vi "CSM Application Running Log Example.vi"() -> ()   [LabVIEW 2017]
doc: "## CSM Application Running Log Example.vi\n\n### Overview\n\nDemonstrates how to use the CSM Logger VIs to implement global CSM event file logging.\n\n### Introduction\n\nThis example demonstrates how to use the CSM Logger VIs to implement global CSM event file logging. Use the CSM-Start File Logger VI, found under LabVIEW Palette -> CSM -> Addons -> Logger, to quickly implement global CSM event file logging.\n\nIn this example, two instances of the CSM-Start File Logger VI are placed in sequence, the log file path and name are manually set , and global rule filters are enabled for each instance separately. After running this example, you can locate and view the corresponding log files to deepen your understanding. If you add/call more CSM modules later, you do not need to change any code here to achieve logging functionality. In summary, a single high-level CSM Addon Logger VI is sufficient to quickly realize a global logging mechanism.\n\n### Steps\n\n- Step1: This is a simple CSM module named `RunningLogExample`.\n- Step2: Any button click will run into the \"API: Button Click\" state and broadcast a status change of the same name, with the button name as the parameter.\n- Step3: In `API: Button Click`, nothing needs to be done because the goal is to observe the log file.\n- Step4: After the program starts, two background logging threads for log files are launched. These logging threads will exit as the program exits.\n- Step5: After running the program, check the directory where the example VI is located for two log files.\n - Step5.1: `CSM Application Running Log Example.csmlog` records all logs.\n - Step5.2: `CSM Application Running Log Example.no-state.csmlog` records logs without state change records."
uses:
  user.lib/_NEVSTOP/Communicable State Machine(CSM)/addons/Logger/CSM File Logger Limit.ctl
  user.lib/_NEVSTOP/Communicable State Machine(CSM)/_Support/Typedef/_CSM_GlobalLog Filter Rules - v1.1.ctl
  user.lib/_NEVSTOP/Communicable State Machine(CSM)/_Support/Typedef/_CSM_GlobalLog_MSG_TYPE.ctl
  user.lib/_NEVSTOP/Communicable State Machine(CSM)/_Support/Typedef/_CSM_GlobalLog_STATE_TYPE.ctl
  user.lib/_NEVSTOP/Communicable State Machine(CSM)/_Support/GlobalEvent/GEvt-Convert Filter Rules - v1.1.vi
  user.lib/_NEVSTOP/Communicable State Machine(CSM)/AdvanceAPI/CSM - Break Down Multiple States String.vi
  user.lib/_NEVSTOP/Communicable State Machine(CSM)/AdvanceAPI/CSM - Compact Multiple States.vi
  user.lib/_NEVSTOP/Communicable State Machine(CSM)/AdvanceAPI/CSM - Revert Arguments-Safe String.vi
  user.lib/_NEVSTOP/Communicable State Machine(CSM)/AdvanceAPI/CSM - Make String Arguments Safe.vi
  user.lib/_NEVSTOP/Communicable State Machine(CSM)/AdvanceAPI/CSM - Keywords.vi
  user.lib/_NEVSTOP/Communicable State Machine(CSM)/_Support/GlobalEvent/LogFilter/SettingVIs/Set Global CSM Filter.vi
  user.lib/_NEVSTOP/Communicable State Machine(CSM)/_Support/GlobalEvent/LogFilter/SettingVIs/Set Global LogType Filter.vi
  user.lib/_NEVSTOP/Communicable State Machine(CSM)/_Support/GlobalEvent/LogFilter/SettingVIs/Set Global State Filter.vi
  user.lib/_NEVSTOP/Communicable State Machine(CSM)/_Support/GlobalEvent/LogFilter/SettingVIs/Set CSM LogType Filter.vi
  user.lib/_NEVSTOP/Communicable State Machine(CSM)/_Support/GlobalEvent/LogFilter/SettingVIs/Set CSM State Filter.vi
  user.lib/_NEVSTOP/Communicable State Machine(CSM)/_Support/GlobalEvent/LogFilter/SettingVIs/Set Global StateType Filter.vi
  user.lib/_NEVSTOP/Communicable State Machine(CSM)/_Support/GlobalEvent/LogFilter/SettingVIs/Set CSM StateType Filter.vi
  user.lib/_NEVSTOP/Communicable State Machine(CSM)/_Support/GlobalEvent/LogFilter/SettingVIs/Set Periodic Log Filter.vi
  user.lib/_NEVSTOP/Communicable State Machine(CSM)/_Shared/Trim Single-line Text.vi
  user.lib/_NEVSTOP/Communicable State Machine(CSM)/_Support/GlobalEvent/LogFilter/LogFilter.lvclass
  user.lib/_NEVSTOP/Communicable State Machine(CSM)/Communicable State Machine.lvlib
  user.lib/_NEVSTOP/Communicable State Machine(CSM)/addons/Logger/CSM File Logger.lvlib
panel:
  in  "Boolean 5":bool
  in  "Boolean 4":bool
  in  "Boolean 3":bool
  in  "Boolean 2":bool
  in  "Boolean 1":bool
  out "State History":string
  # "#CSM-Example Overview\n\nDemonstrates how to use the CSM Logger VIs to implement global CSM event file logging."
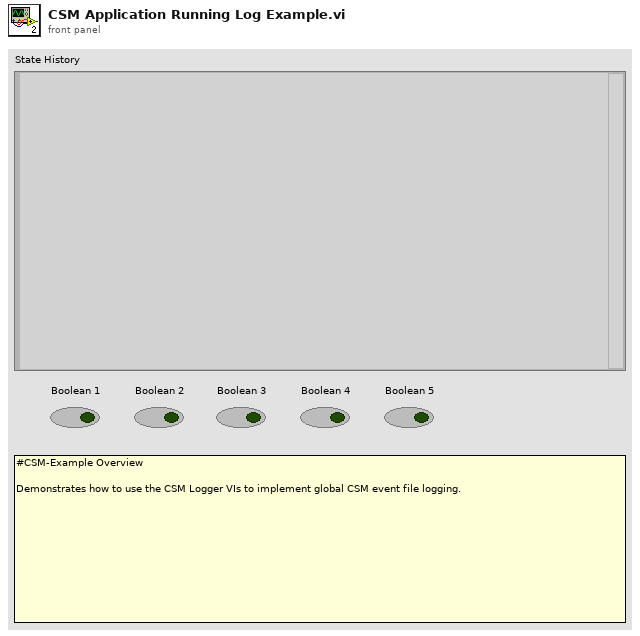
[diagram p1: front panel]
types:
  T1 = typedef "Communicable State Machine.lvlib/_CSM_GlobalLog Filter Rules - v1.1.ctl" = cluster{"Global":cluster{"CSM":string[], "LogType":T2[], "State":string[], "StateType":T3[]}, "CSM":cluster{"LogType":cluster{"CSM":string, "LogType":T2}[], "State":cluster{"CSM":string, "State":string}[], "StateType":cluster{"CSM":string, "LogType":T3}[]}, "PeriodicMessageFilter":cluster{"Enable":bool, "Threshold(#/s)":dbl, "CheckPeriod(s)":dbl}}
  T2 = typedef "Communicable State Machine.lvlib/_CSM_GlobalLog_MSG_TYPE.ctl" = enum16{"User Log", "State Change", "Status", "Interrupt", "Register", "Unregister", "Error Log", "Module Created", "Module Destroyed"}
  T3 = typedef "Communicable State Machine.lvlib/_CSM_GlobalLog_STATE_TYPE.ctl" = enum16{"State - Internal State", "State - External Message", "State - Response", "State - Complete"}
  T4 = typedef "CSM File Logger.lvlib/CSM File Logger Limit.ctl" = cluster{"file size (in bytes)":i64, "file num":i32}
  T5 = enum32{"Invalid", "Standard", "Closed", "Hidden", "Minimized", "Maximized"}
  T6 = enum32{"invalid app kind", "Development System", "Run Time System", "Student Edition", "Embedded LabVIEW", "Evaluation", "Custom"}
  T7 = typedef "Communicable State Machine.lvlib/_CSM_Response Source Message.ctl" = cluster{"‘State":string, "’Arguments":string, "’Error":errorcluster}
  T8 = cluster{"Current VI Reference":refnum<vi>, "Close Panel on Exit?":bool}
  T9 = cluster{"Core":cluster{"Current VI Reference":refnum<vi>, "Close Panel on Exit?":bool}, "Your Boolean data":bool, "Your string data":string}
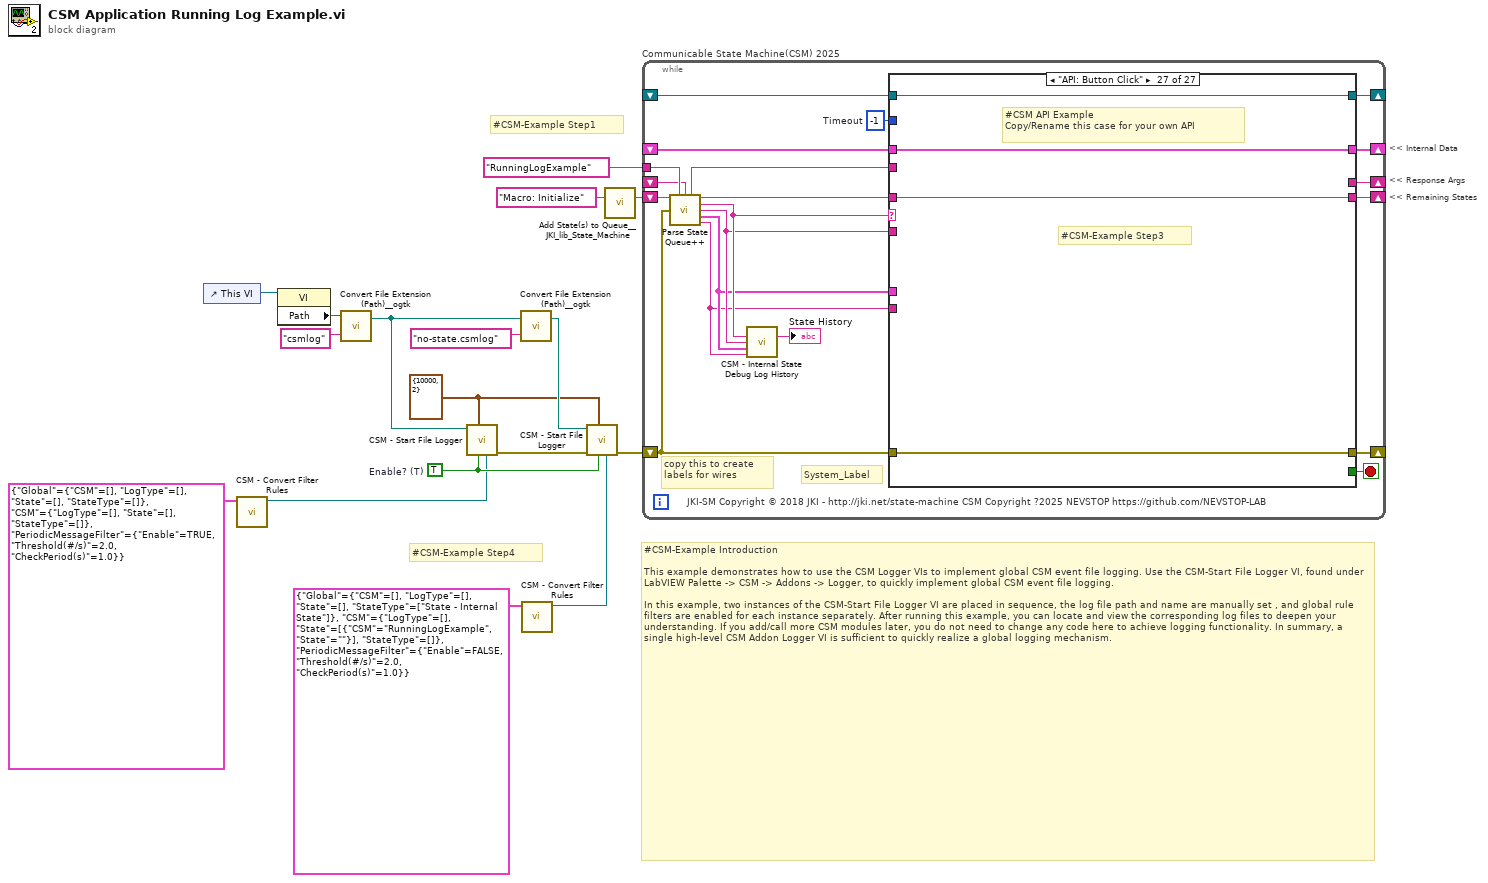
[diagram p0: block diagram]
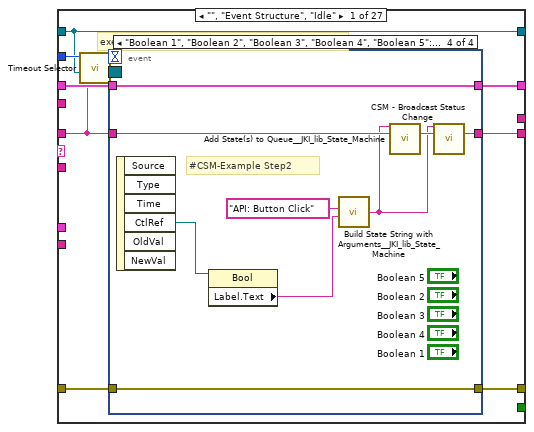
[diagram p2: hidden frame]
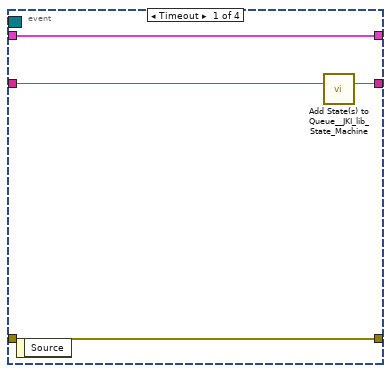
[diagram p3: hidden frame]
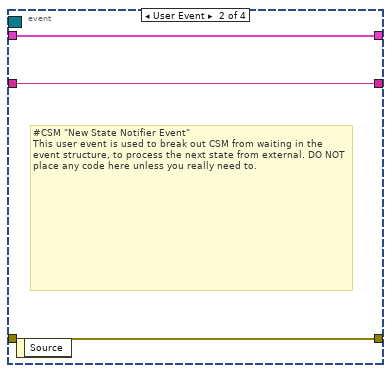
[diagram p4: hidden frame]
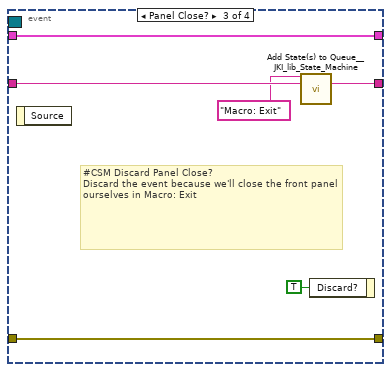
[diagram p5: hidden frame]
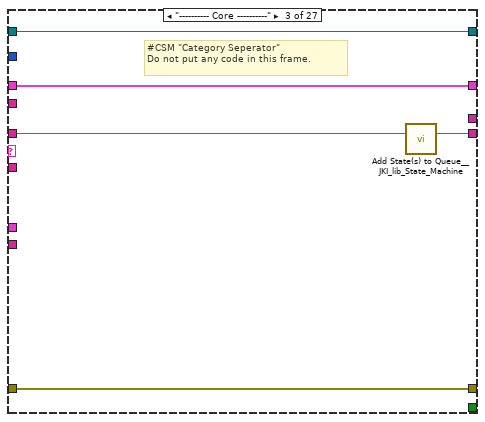
[diagram p7: hidden frame]
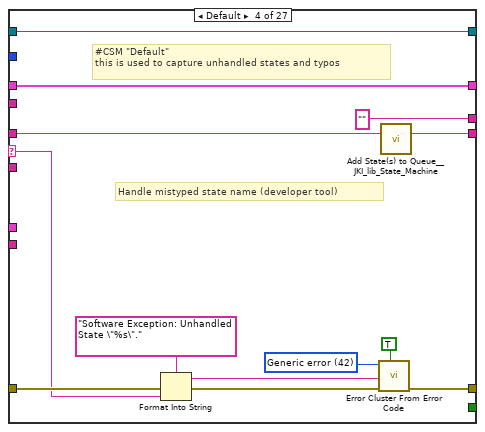
[diagram p8: hidden frame]
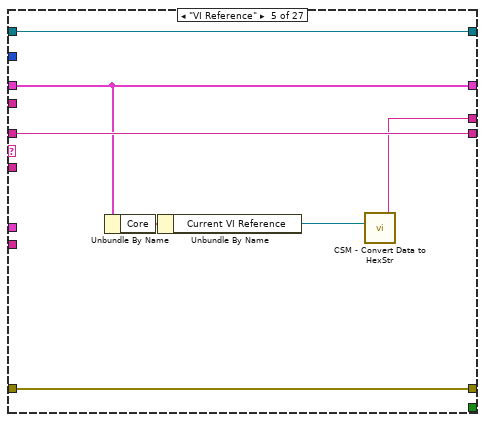
[diagram p9: hidden frame]
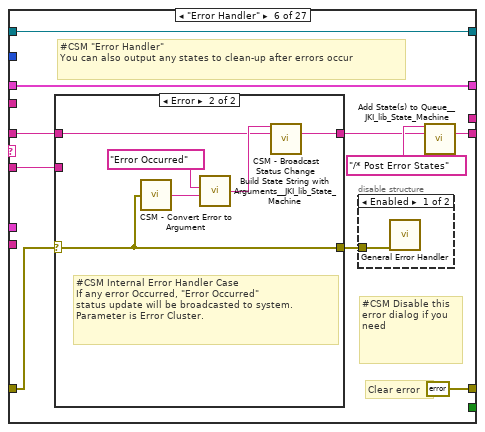
[diagram p10: hidden frame]
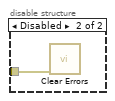
[diagram p11: hidden frame]
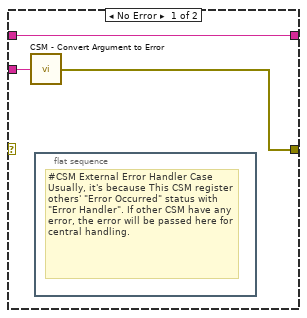
[diagram p12: hidden frame]
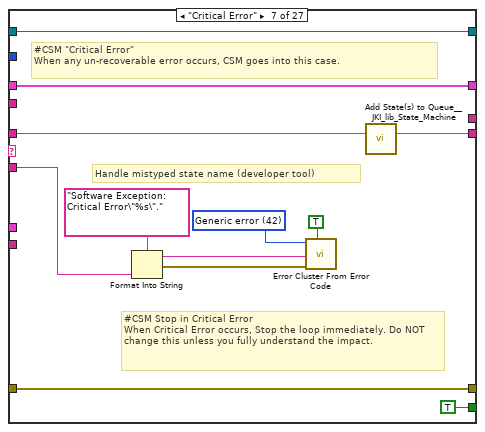
[diagram p13: hidden frame]
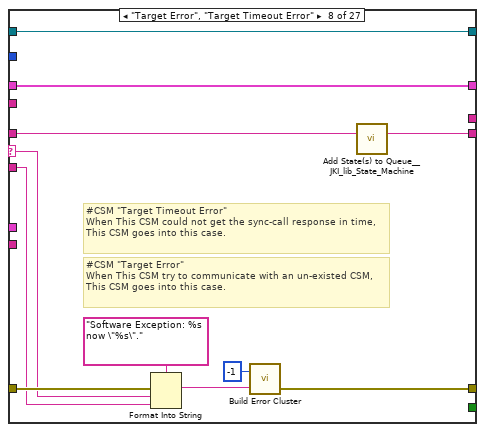
[diagram p14: hidden frame]
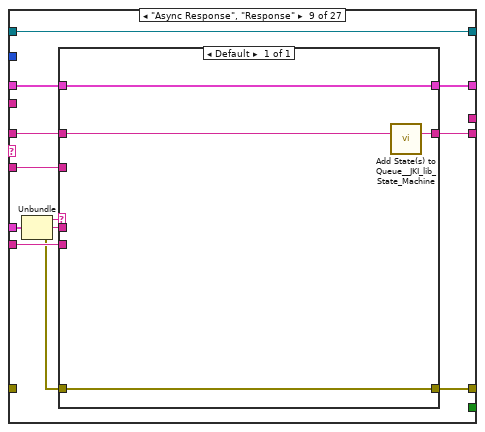
[diagram p15: hidden frame]
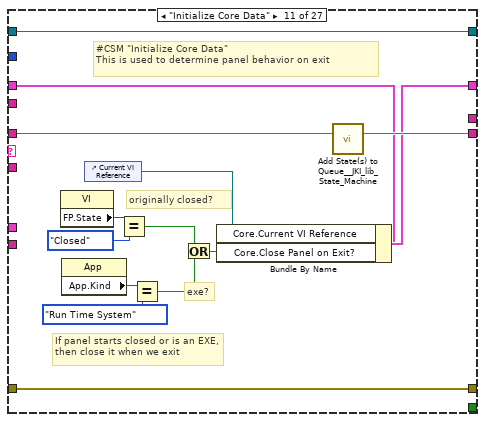
[diagram p17: hidden frame]
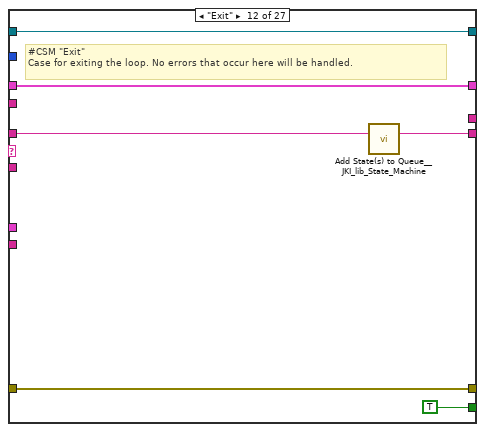
[diagram p18: hidden frame]
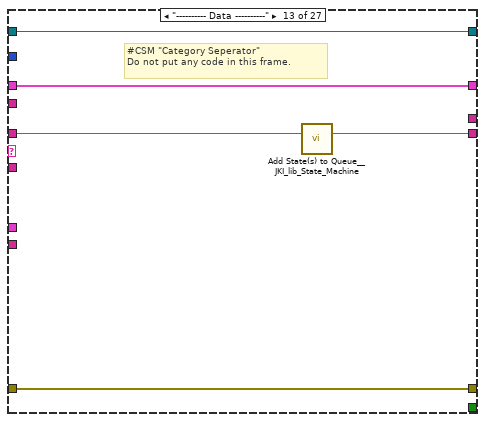
[diagram p19: hidden frame]
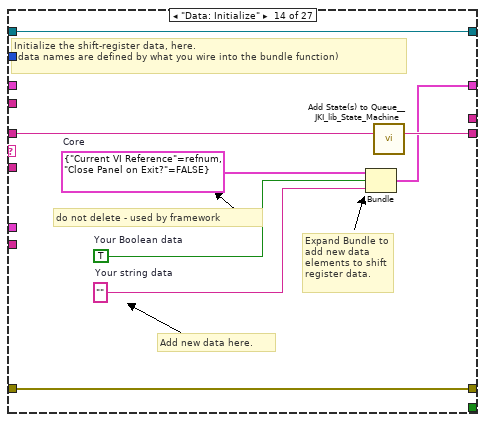
[diagram p20: hidden frame]
diagram:
  w5 = T4 {"file size (in bytes)"=10000, "file num"=2} ("log limit")
  w9 = TRUE  # Enable? (T)
  # "#CSM-Example Step4"
  # "#CSM-Example Step1"
  # "#CSM-Example Introduction\n\nThis example demonstrates how to use the CSM Logger VIs to implement global CSM event file logging. Use the CSM-Start File Logger VI, found under LabVIEW Palette -> CSM -> Addons -> Logger, to quickly implement global CSM event file logging.\n\nIn this example, two instances of the CSM-Start File Logger VI are placed in sequence, the log file path and name are manually set , and global rule filters are enabled for each instance separately. After running this example, you can locate and view the corresponding log files to deepen your understanding. If you add/call more CSM modules later, you do not need to change any code here to achieve logging functionality. In summary, a single high-level CSM Addon Logger VI is sufficient to quickly realize a global logging mechanism."
  # "<< Internal Data"
  # "<< Response Args"
  # "<< Remaining States"
  n1 = control-ref of="This VI"() -> (w13:refnum<vi>)
  n2 = call-poly "CSM - Convert Filter Rules.vi"("Rules-v1"=T1 {"Global"={"CSM"=[], "LogType"=[], "State"=[], "StateType"=[]}, "CSM"={"LogType"=[], "State"=[], "StateType"=[]}, "PeriodicMessageFilter"={"Enable"=TRUE, "Threshold(#/s)"=2.0, "CheckPeriod(s)"=1.0}}) -> ("GlobalLogFilter"=w1:refnum<class "LogFilter.lvclass">)  [unwired: 10 in]
  n3 = property class="VI"(reference=w13) -> ("Path"=w12:path)  [unwired: 1 in, 2 out]
  n4 = call "Convert File Extension (Path)__ogtk.vi"("New Ending (None)"="csmlog" ("new ending (none)"), "File Name"=w12) -> ("New Filename"=w7:path)  [unwired: 1 out]
  n5 = call "CSM - Start File Logger.vi"("Filter Rules"=w1, "Enable? (T)"=w9, "Log Limit"=w5, "Log File Path"=w7) -> ("error out"=w10:errorcluster)  [unwired: 5 in, 2 out]
  n6 = call "Convert File Extension (Path)__ogtk.vi"("New Ending (None)"="no-state.csmlog" ("new ending (none)"), "File Name"=w7) -> ("New Filename"=w6:path)  [unwired: 1 out]
  n7 = call-poly "CSM - Convert Filter Rules.vi"("Rules-v1"=T1 {"Global"={"CSM"=[], "LogType"=[], "State"=[], "StateType"=[enum."State - Internal State"]}, "CSM"={"LogType"=[], "State"=[{"CSM"="RunningLogExample", "State"=""}], "StateType"=[]}, "PeriodicMessageFilter"={"Enable"=FALSE, "Threshold(#/s)"=2.0, "CheckPeriod(s)"=1.0}}) -> ("GlobalLogFilter"=w4:refnum<class "LogFilter.lvclass">)  [unwired: 10 in]
  n8 = call "CSM - Start File Logger.vi"("Filter Rules"=w4, "Enable? (T)"=w9, "Log Limit"=w5, "Error In"=w10, "Log File Path"=w6) -> ("error out"=w14:errorcluster)  [unwired: 4 in, 2 out]
  n9 = call <vilib>:"Add State(s) to Queue__JKI_lib_State_Machine.vi"("State(s) in (\"\")"="Macro: Initialize" ("Init State(\"Macro: Initialize\")")) -> ("States Out"=w15:string)  [unwired: 14 in]
  n10 = while "Communicable State Machine(CSM) 2025" {
    shift-right: [w32] -> _
    shift-left: _ -> [w31]
    shift-right: [w35] -> _
    shift-left: w14 -> [w29]
    shift-right: [w34] -> _
    shift-left: w15 -> [w36]
    tunnel: "RunningLogExample" ("Name (\"\" to Use UUID)") -> [w25]
    shift-right: [w28] -> _
    shift-left: _ -> [w19]
    shift-right: [w27] -> _
    shift-left: _ -> [w26]
    stop <- w33 stop-if-true
    w30 = -1  # Timeout
    # "copy this to create labels for wires"
    # "System_Label"
    # "JKI-SM Copyright © 2018 JKI - http://jki.net/state-machine CSM Copyright ?2025 NEVSTOP https://github.com/NEVSTOP-LAB"
    n11 = call "Parse State Queue++.vi"("State Queue"=w36, "Name (\"\" to Use UUID)"=w25, "Response Arguments"=w19, "Previous Error"=w29) -> ("Name Used"=w20:string, "Remaining States"=w37:string, "Current State"=w24:string, "Arguments"=w23:string, "Additional Information"=w22:T7, "Source CSM"=w21:string)  [unwired: 6 in]
    n12 = call "CSM - Internal State Debug Log History.vi"("State"=w24, "Arguments (\"\")"=w23, ">> Response Source Message >>"=w22, "Source (\"\")"=w21) -> ("Debug Log"=→"State History":string)  [unwired: 11 in]
    n13 = case shown="\"API: Button Click\"" w24 {
      selector: w24 -> [_ _ _ w80 _ _ _ w134 _ _ _ _ _ _ _ _ _ _ _ _ _ _ _ _ _ _ _]
      tunnel: w37 -> [w38 w71 w77 w84 w96 w102 w128 w136 w147 w160 w175 w181 w186 w194 w201 w206 w213 w217 w223 w228 w235 w251 w321 w327 w339 w342 w346]
      tunnel: w23 -> [_ _ _ _ _ w101 w121 w135 w146 _ _ _ _ _ _ _ _ _ _ _ w230 w245 _ _ _ _ _]
      tunnel: w31 -> [w45 w70 w74 w82 w95 w106 w129 w138 w149 w159 w168 w179 w183 _ w196 w203 w212 w216 w220 w226 w233 w247 w318 w324 w336 w341 w345]
      tunnel: [w44 w72 w75 w86 w97 errorcluster {"status"=FALSE, "code"=0, "source"=""} ("error out") w130 w132 w152 w161 w172 w178 w184 w191 w197 w204 w207 w215 w221 w225 w231 w248 w319 w325 w337 w343 w347] -> w35
      tunnel: w29 -> [w43 w72 w75 w85 w97 w103 w130 w140 _ w161 w172 w178 w184 w191 w198 w204 _ w218 w221 w225 w232 w249 w319 w325 w337 w343 w347]
      tunnel: [w46 w71 w76 w83 w96 w98 w127 w139 w148 w160 w174 w180 w185 w193 w200 w205 w213 w217 w222 w227 w234 w250 w320 w326 w338 w342 w346] -> w34
      tunnel: [_ _ _ _ _ _ TRUE _ _ _ _ TRUE _ _ _ _ _ _ _ _ _ _ _ _ _ _ _] -> w33
      tunnel: [w42 w70 w74 w82 w95 w106 w129 w138 w150 w159 w173 w179 w183 w192 w196 w203 w212 w216 w220 w226 w233 w247 w318 w324 w336 w341 w345] -> w32
      tunnel: w30 -> [w41 _ _ _ _ _ _ _ _ _ _ _ _ _ _ _ _ _ _ _ _ _ _ _ _ _ _]
      tunnel: w21 -> [_ _ _ _ _ _ _ _ w144 _ _ _ _ _ _ _ _ _ _ _ _ _ _ _ _ _ _]
      tunnel: w22 -> [_ _ _ _ _ _ _ _ w151 _ _ _ _ _ _ _ _ _ _ _ _ _ _ _ _ _ _]
      tunnel: [_ _ _ "" w91 _ _ _ _ _ _ _ _ _ _ _ _ _ _ _ _ _ _ _ _ _ _] -> w28
      tunnel: [w40 w69 w73 w78 w94 w105 w119 w137 w153 w158 w162 w176 w182 w187 w195 w202 w211 w214 w219 w224 w229 w244 w317 w322 w329 w340 w344] -> w27
      tunnel: w26 -> [w40 w69 w73 w78 w94 w105 w119 w137 w153 w158 w162 w176 w182 w187 w195 w202 _ w214 w219 w224 w229 w244 w317 w322 w329 w340 w344]
      tunnel: w20 -> [_ _ _ _ _ _ _ _ _ _ _ _ _ _ _ _ w210 _ _ _ _ _ _ _ _ _ _]
      frame "", "Event Structure", "Idle" {
        # "executes when the state queue is empty"
        n14 = call "Timeout Selector.vi"("Remaining States"=w38, "Timeout Expected"=w41) -> ("Timeout"=w39:i32)  [unwired: 5 in]
        n15 = event shown="[3] \"Boolean 1\", \"Boolean 2\", \"Boolean 3\", \"Boolean 4\", \"Boolean 5\": Value Change" {
          selector: w40 -> [_ _ _ _]
          dyn-events: _ -> [_ _ _ _]
          timeout: w39 -> [_ _ _ _]
          tunnel: w38 -> [w50 w52 w59 w66]
          tunnel: [w49 w52 w58 w61] -> w46
          tunnel: w45 -> [w47 w53 w56 w67]
          tunnel: [w48 w51 w57 w68] -> w44
          tunnel: w43 -> [w48 w51 w57 w68]
          tunnel: [w47 w53 w56 w67] -> w42
          event Timeout {
            n16 = event-data() -> ()  [unwired: 1 in, 1 out]
            n17 = call <vilib>:"Add State(s) to Queue__JKI_lib_State_Machine.vi"("State(s) in (\"\")"=w50) -> ("States Out"=w49:string)  [unwired: 14 in]
          }
          event User Event {
            # "#CSM \"New State Notifier Event\"\nThis user event is used to break out CSM from waiting in the event structure, to process the next state from external. DO NOT place any code here unless you really need to."
            n18 = event-data() -> ()  [unwired: 1 in, 1 out]
          }
          event Panel Close? {
            # "#CSM Discard Panel Close?\nDiscard the event because we'll close the front panel ourselves in Macro: Exit"
            n19 = event-data() -> ()  [unwired: 1 in, 1 out]
            n20 = call <vilib>:"Add State(s) to Queue__JKI_lib_State_Machine.vi"("State(s) in Front (\"\")"="Macro: Exit", "State(s) in (\"\")"=w59) -> ("States Out"=w58:string)  [unwired: 13 in]
            n21 = event-data("Discard?"=TRUE) -> ()  [unwired: 1 in, 1 out]
          }
          event "Boolean 1", "Boolean 2", "Boolean 3", "Boolean 4", "Boolean 5": Value Change {
            # "#CSM-Example Step2"
            n22 = event-data() -> ("CtlRef"=w63:refnum<vi>)  [unwired: 1 in, 5 out]
            n23 = property class="Bool"(reference=w63) -> ("Label.Text"=w62:string)  [unwired: 1 in, 2 out]
            n24 = call <vilib>:"Build State String with Arguments__JKI_lib_State_Machine.vi"("Arguments (\"\")"=w62, "State"="API: Button Click") -> ("State with Arguments"=w60:string)  [unwired: 4 in]
            n25 = call <vilib>:"Add State(s) to Queue__JKI_lib_State_Machine.vi"("State(s) in Front (\"\")"=w60, "State(s) in (\"\")"=w66) -> ("States Out"=w65:string)  [unwired: 13 in]
            n26 = call "CSM - Broadcast Status Change.vi"("Status With Arguments"=w60, "State Queue"=w65) -> ("Remaining States"=w61:string)  [unwired: 13 in]
          }
        }
      }
      frame "CSM Documentation" {
        # "#CSM README FIRST\n\nCSM is a LabVIEW application framework that builds upon JKI State Machine (JKISM). It follows the pattern of JKISM and extends the keywords to describe message communication between CSM modules, including concepts such as Sync-Message, Async-Message, Subscription/Unsubscription of status - essential elements for creating reusable code modules. For more information, please visit the CSM wiki: https://github.com/NEVSTOP-LAB/JKI-State-Machine-Plus-Plus/wiki\n\nFor instructions on JKI State Machine, visit: http://jki.net/state-machine/\nFor information about CSM, visit: https://github.com/NEVSTOP-LAB"
        # "#CSM \"Documentation\"\nCase for holding CSM Documenation"
      }
      frame "---------- Core ----------" {
        # "#CSM \"Category Seperator\"\nDo not put any code in this frame."
        n27 = call <vilib>:"Add State(s) to Queue__JKI_lib_State_Machine.vi"("State(s) in (\"\")"=w77) -> ("States Out"=w76:string)  [unwired: 14 in]
      }
      frame Default {
        w89 = 42 items=["No error", "Argument error", "Memory is full", "Out of zone", "End of file", "File already open", "Generic file I/O error", "File not found", "File permission error", "Disk is full", "Duplicate path", "Too many files open", "System feature not enabled", "Resource file not found", "Cannot add resource", "Resource not found", "Image not found", "Image memory error", "Pen does not exist", "Config type invalid", "Config token not found", "Config parse error", "Config memory error", "Bad external code format", "Bad external code offset", "External code not present", "Null window", "Destroy window error", "Null menu", "Print aborted", "Bad print record", "Print driver error", "Windows error during printing", "Memory error during printing", "Print dialog error", "Generic print error", "Invalid device refnum", "Device not found", "Device parameter error", "Device unit error", "Cannot open device", "Device call aborted", "Generic error", "Cancelled by user", "Object ID too low", "Object ID too high", "Object not in heap", "Unknown heap", "Unknown object (invalid DefProc)", "Unknown object (DefProc not in table)", "Message out of range", "Invalid (null) method", "Unknown message", "Manager call not supported", "Bad address", "Network operation in progress", "Network operation timed out", "Connection is busy", "Network attribute not supported", "Network error", "Address in use", "System out of memory", "Connection aborted", "Connection refused", "Not connected", "Already connected", "Connection closed", "Initialization error (interapplication manager)", "Bad occurrence", "Wait on unbound occurrence handler", "Occurrence queue overflow", "Datalog type conflict", "Unused", "Unrecognized type (interapplication manager)", "Memory corrupt", "Failed to make temporary DLL", "Old CIN version", "Drag socket not found", "Failed to load drop-object", "Failed to register OLE object", "Failed to release OLE object", "Format specifier type mismatch", "Unknown format specifier", "Too few format specifiers", "Too many format specifiers", "Scan failed", "Newer CIN version", "Error converting to variant", "Runtime menu error", "Password tampered", "Variant attribute not found", "Incompatible variant data type", "Event data is not available", "Event Store is not present", "Occurrence is not found", "Event Queue is not created", "Event info is not available", "Refnum passed is NULL", "Error retrieving Class GUID", "Error retrieving CoClass GUID", "Error retrieving TypeLib GUID.", "Bad built application magic bytes.", "Specific driver is different from the specific driver associated with the Logical Name.", "There is no session opened to the class driver.", "Max Error", "MAX - Error with config objects", "MAX - Error loading configuration", "MAX - Group not supported"]
        # "#CSM \"Default\"\nthis is used to capture unhandled states and typos"
        # "Handle mistyped state name (developer tool)"
        n28 = Format Into String(format string="Software Exception: Unhandled State \"%s\"." ("message"), error in=w85, w80) -> (resulting string=w88:string, error out=w87:errorcluster)  [unwired: 1 in]
        n29 = call <vilib>:"Error Cluster From Error Code.vi"("show call chain? (False)"=TRUE, "error in (no error)"=w87, "error message (\"\")"=w88, "error code (0)"=w89) -> ("error out"=w86:errorcluster)  [unwired: 5 in]
        n30 = call <vilib>:"Add State(s) to Queue__JKI_lib_State_Machine.vi"("State(s) in (\"\")"=w84) -> ("States Out"=w83:string)  [unwired: 14 in]
      }
      frame "VI Reference" {
        n31 = Unbundle By Name(w95) -> ("Core"=w93:T8)
        n32 = Unbundle By Name(w93) -> ("Current VI Reference"=w92:refnum<vi>)
        n33 = call "CSM - Convert Data to HexStr.vi"("Variant"=w92) -> ("HEX String (0-9,A-F)"=w91:string)  [unwired: 8 in]
      }
      frame "Error Handler" {
        # "#CSM Disable this error dialog if you need"
        # "#CSM \"Error Handler\"\nYou can also output any states to clean-up after errors occur"
        # "Clear error"
        n34 = case shown="Error" w103 {
          selector: w103 -> [_ w113]
          tunnel: [w112 w115] -> w99
          tunnel: w102 -> [w112 w114]
          tunnel: w101 -> [w111 _]
          tunnel: [w110 w113] -> w104
          frame No Error {
            n35 = call "CSM - Convert Argument to Error.vi"("Argument"=w111) -> ("Error"=w110:errorcluster)  [unwired: 4 in]
            n36 = flat-sequence {
              frame #0 {
                # "#CSM External Error Handler Case\nUsually, it's because This CSM register others' \"Error Occurred\" status with \"Error Handler\". If other CSM have any error, the error will be passed here for central handling."
              }
            }
          }
          frame Error {
            # "#CSM Internal Error Handler Case \nIf any error Occurred, \"Error Occurred\" \nstatus update will be broadcasted to system.\nParameter is Error Cluster."
            n37 = call "CSM - Convert Error to Argument.vi"("Error"=w113) -> ("Argument"=w117:string)  [unwired: 4 in]
            n38 = call <vilib>:"Build State String with Arguments__JKI_lib_State_Machine.vi"("Arguments (\"\")"=w117, "State"="Error Occurred" ("Status with Arguments")) -> ("State with Arguments"=w116:string)  [unwired: 4 in]
            n39 = call "CSM - Broadcast Status Change.vi"("Status With Arguments"=w116, "State Queue"=w114) -> ("Remaining States"=w115:string)  [unwired: 13 in]
          }
        }
        n40 = disable-structure shown="Enabled" {
          disable-tunnel: w104 -> [w108 w109]
          frame Enabled {
            n41 = call <vilib>:"General Error Handler.vi"("error in (no error)"=w108) -> ()  [unwired: 10 in, 5 out]
          }
          frame Disabled {
            n42 = call <vilib>:"Clear Errors.vi"("error in (no error)"=w109) -> ()  [unwired: 5 in, 2 out]
          }
        }
        n43 = call <vilib>:"Add State(s) to Queue__JKI_lib_State_Machine.vi"("State(s) in Front (\"\")"="/* Post Error States", "State(s) in (\"\")"=w99) -> ("States Out"=w98:string)  [unwired: 13 in]
      }
      frame "Critical Error" {
        w125 = 42 items=["No error", "Argument error", "Memory is full", "Out of zone", "End of file", "File already open", "Generic file I/O error", "File not found", "File permission error", "Disk is full", "Duplicate path", "Too many files open", "System feature not enabled", "Resource file not found", "Cannot add resource", "Resource not found", "Image not found", "Image memory error", "Pen does not exist", "Config type invalid", "Config token not found", "Config parse error", "Config memory error", "Bad external code format", "Bad external code offset", "External code not present", "Null window", "Destroy window error", "Null menu", "Print aborted", "Bad print record", "Print driver error", "Windows error during printing", "Memory error during printing", "Print dialog error", "Generic print error", "Invalid device refnum", "Device not found", "Device parameter error", "Device unit error", "Cannot open device", "Device call aborted", "Generic error", "Cancelled by user", "Object ID too low", "Object ID too high", "Object not in heap", "Unknown heap", "Unknown object (invalid DefProc)", "Unknown object (DefProc not in table)", "Message out of range", "Invalid (null) method", "Unknown message", "Manager call not supported", "Bad address", "Network operation in progress", "Network operation timed out", "Connection is busy", "Network attribute not supported", "Network error", "Address in use", "System out of memory", "Connection aborted", "Connection refused", "Not connected", "Already connected", "Connection closed", "Initialization error (interapplication manager)", "Bad occurrence", "Wait on unbound occurrence handler", "Occurrence queue overflow", "Datalog type conflict", "Unused", "Unrecognized type (interapplication manager)", "Memory corrupt", "Failed to make temporary DLL", "Old CIN version", "Drag socket not found", "Failed to load drop-object", "Failed to register OLE object", "Failed to release OLE object", "Format specifier type mismatch", "Unknown format specifier", "Too few format specifiers", "Too many format specifiers", "Scan failed", "Newer CIN version", "Error converting to variant", "Runtime menu error", "Password tampered", "Variant attribute not found", "Incompatible variant data type", "Event data is not available", "Event Store is not present", "Occurrence is not found", "Event Queue is not created", "Event info is not available", "Refnum passed is NULL", "Error retrieving Class GUID", "Error retrieving CoClass GUID", "Error retrieving TypeLib GUID.", "Bad built application magic bytes.", "Specific driver is different from the specific driver associated with the Logical Name.", "There is no session opened to the class driver.", "Max Error", "MAX - Error with config objects", "MAX - Error loading configuration", "MAX - Group not supported"]
        # "#CSM Stop in Critical Error\nWhen Critical Error occurs, Stop the loop immediately. Do NOT change this unless you fully understand the impact."
        # "#CSM \"Critical Error\"\nWhen any un-recoverable error occurs, CSM goes into this case."
        # "Handle mistyped state name (developer tool)"
        n44 = Format Into String(format string="Software Exception: Critical Error\"%s\"." ("message"), w121) -> (resulting string=w124:string, error out=w123:errorcluster)  [unwired: 2 in]
        n45 = call <vilib>:"Error Cluster From Error Code.vi"("show call chain? (False)"=TRUE, "error in (no error)"=w123, "error message (\"\")"=w124, "error code (0)"=w125) -> ()  [unwired: 5 in, 1 out]
        n46 = call <vilib>:"Add State(s) to Queue__JKI_lib_State_Machine.vi"("State(s) in (\"\")"=w128) -> ("States Out"=w127:string)  [unwired: 14 in]
      }
      frame "Target Error", "Target Timeout Error" {
        # "#CSM \"Target Error\"\nWhen This CSM try to communicate with an un-existed CSM, This CSM goes into this case."
        # "#CSM \"Target Timeout Error\"\nWhen This CSM could not get the sync-call response in time, This CSM goes into this case."
        n47 = Format Into String(format string="Software Exception: %s now \"%s\"." ("message"), error in=w140, w134, w135) -> (resulting string=w133:string)  [unwired: 1 in, 1 out]
        n48 = call "Build Error Cluster.vi"("String to Prepend to Source (\"\")"=w133, "Code"=-1 ("code")) -> ("error out"=w132:errorcluster)
        n49 = call <vilib>:"Add State(s) to Queue__JKI_lib_State_Machine.vi"("State(s) in (\"\")"=w136) -> ("States Out"=w139:string)  [unwired: 14 in]
      }
      frame "Async Response", "Response" {
        n50 = Unbundle(w151) -> ("‘State"=w145:string, "’Arguments"=w143:string, "’Error"=w142:errorcluster)
        n51 = case shown="Default" w145 {
          tunnel: [w157] -> w152
          tunnel: w142 -> [w157]
          tunnel: [w156] -> w150
          tunnel: w149 -> [w156]
          tunnel: [w154] -> w148
          tunnel: w147 -> [w155]
          tunnel: w146 -> [_]
          tunnel: w144 -> [_]
          tunnel: w143 -> [_]
          frame Default {
            n52 = call <vilib>:"Add State(s) to Queue__JKI_lib_State_Machine.vi"("State(s) in (\"\")"=w155) -> ("States Out"=w154:string)  [unwired: 14 in]
          }
        }
      }
      frame "Async Message Posted" {
        # "#CSM \"Async Message Posted\"\nAfter Async Message is posted (-> or ->| ), CSM goes to this state for post-action.\nYou can use Argument - State to tell which Async Message is called."
      }
      frame "Initialize Core Data" {
        # "#CSM \"Initialize Core Data\"\nThis is used to determine panel behavior on exit"
        # "originally closed?"
        # "exe?"
        # "If panel starts closed or is an EXE, then close it when we exit"
        n53 = property class="VI"() -> ("FP.State"=w165:T5)  [unwired: 2 in, 2 out]
        n54 = property class="App"() -> ("App.Kind"=w171:T6)  [unwired: 2 in, 2 out]
        n55 = control-ref of="Current VI Reference"() -> (w166:refnum<vi>)
        n56 = Equal?(x=w165, y=T5."Closed" ("Front Panel Window:State")) -> (x = y?=w163:bool)
        n57 = Equal?(x=w171, y=T6."Run Time System" ("Application:Kind")) -> (x = y?=w169:bool)
        n58 = Or(x=w163, y=w169) -> (x .or. y?=w167:bool)
        n59 = Bundle By Name(cluster=w168, "Core.Current VI Reference"=w166, "Core.Close Panel on Exit?"=w167) -> (w173:T9)
        n60 = call <vilib>:"Add State(s) to Queue__JKI_lib_State_Machine.vi"("State(s) in (\"\")"=w175) -> ("States Out"=w174:string)  [unwired: 14 in]
      }
      frame "Exit" {
        # "#CSM \"Exit\"\nCase for exiting the loop. No errors that occur here will be handled."
        n61 = call <vilib>:"Add State(s) to Queue__JKI_lib_State_Machine.vi"("State(s) in (\"\")"=w181) -> ("States Out"=w180:string)  [unwired: 14 in]
      }
      frame "---------- Data ----------" {
        # "#CSM \"Category Seperator\"\nDo not put any code in this frame."
        n62 = call <vilib>:"Add State(s) to Queue__JKI_lib_State_Machine.vi"("State(s) in (\"\")"=w186) -> ("States Out"=w185:string)  [unwired: 14 in]
      }
      frame "Data: Initialize" {
        w188 = T8 {"Current VI Reference"=refnum, "Close Panel on Exit?"=FALSE}  # Core
        w190 = TRUE  # Your Boolean data
        w189 = ""  # Your string data
        # "do not delete - used by framework"
        # "Expand Bundle to add new data elements to shift register data."
        # "Add new data here."
        # "Initialize the shift-register data, here.\n(data names are defined by what you wire into the bundle function)"
        n63 = Bundle("Core"=w188, "Your Boolean data"=w190, "Your string data"=w189) -> (w192:T9)  [unwired: 1 in]
        n64 = call <vilib>:"Add State(s) to Queue__JKI_lib_State_Machine.vi"("State(s) in (\"\")"=w194) -> ("States Out"=w193:string)  [unwired: 14 in]
      }
      frame "Data: Cleanup" {
        # "Cleanup any data and references, here.\n(this is called automatically, by the Macro: Exit)"
        n65 = Unbundle By Name(w196) -> ("Core.Current VI Reference"=w199:refnum<vi>)
        n66 = Close Reference(reference=w199, error in (no error)=w198) -> (error out=w197:errorcluster)
        n67 = call <vilib>:"Add State(s) to Queue__JKI_lib_State_Machine.vi"("State(s) in (\"\")"=w201) -> ("States Out"=w200:string)  [unwired: 14 in]
      }
      frame "---------- Events ----------" {
        # "#CSM \"Category Seperator\"\nDo not put any code in this frame."
        n68 = call <vilib>:"Add State(s) to Queue__JKI_lib_State_Machine.vi"("State(s) in (\"\")"=w206) -> ("States Out"=w205:string)  [unwired: 14 in]
      }
      frame "Events: Register" {
        # "#CSM \"Events: Register\"\nRegister user event. New Message Event is registered to break CSM waiting in event structure by default."
        # "#CSM Register New Message Event\nRegister message event to break Waiting in Event structure."
        n69 = call "CSM - Get New State Notifier Event.vi"("Name (\"\" to Use UUID)"=w210) -> ("error out"=w208:errorcluster, "New State Notifier Event"=w209:refnum<user-event>)  [unwired: 9 in]
        n70 = register-events(error in=w208, w209) -> (reference out=w211:refnum<event-registration>, error out=w207:errorcluster)  [unwired: 1 in]
      }
      frame "Events: Unregister" {
        # "#CSM \"Events: Unregister\"\nUnregister user event."
        n71 = Unregister For Events(event registration refnum=w214, error in=w218) -> (error out=w215:errorcluster)
      }
      frame "---------- UI ----------" {
        # "#CSM \"Category Seperator\"\nDo not put any code in this frame."
        n72 = call <vilib>:"Add State(s) to Queue__JKI_lib_State_Machine.vi"("State(s) in (\"\")"=w223) -> ("States Out"=w222:string)  [unwired: 14 in]
      }
      frame "UI: Initialize" {
        # "#CSM \"UI: Initialize\"\nInitialize the User Interface, here.\n(this is called automatically, by the Macro: Init)"
        n73 = call <vilib>:"Add State(s) to Queue__JKI_lib_State_Machine.vi"("State(s) in (\"\")"=w228) -> ("States Out"=w227:string)  [unwired: 14 in]
      }
      frame "UI: Cursor Set" {
        # "#CSM \"UI: Cursor Set\"\nSet and Unset Cursor Busy.\n(Usage: \"UI: Cursor Set >> Busy|Idle\")"
        # "Argument"
        n74 = disable-structure shown="TARGET_TYPE!=Windows" {
          disable-tunnel: w232 -> [w238 w243]
          disable-tunnel: [w237 w243] -> w231
          disable-tunnel: w230 -> [w236 _]
          frame condition #0 (active) {
            n75 = case shown="\"Idle\", Default" w236 {
              tunnel: w238 -> [w240 w242]
              tunnel: [w239 w241] -> w237
              frame "Idle", Default {
                n76 = call <vilib>:"Unset Busy.vi"("error in (no error)"=w240) -> ("error out"=w239:errorcluster)  [unwired: 10 in]
              }
              frame "Busy" {
                n77 = call <vilib>:"Set Busy.vi"("error in (no error)"=w242) -> ("error out"=w241:errorcluster)  [unwired: 9 in, 1 out]
              }
            }
          }
          frame condition #1 {
          }
        }
        n78 = call <vilib>:"Add State(s) to Queue__JKI_lib_State_Machine.vi"("State(s) in (\"\")"=w235) -> ("States Out"=w234:string)  [unwired: 14 in]
      }
      frame "UI: Front Panel State" {
        # "#CSM \"UI: Front Panel State\"\nSet Front Panel Open or Closed\n(Usage: \"UI: Front Panel State >> Open|Close\")"
        # "Argument"
        n79 = Unbundle By Name(w247) -> ("Core.Current VI Reference"=w246:refnum<vi>)
        n80 = call <vilib>:"Add State(s) to Queue__JKI_lib_State_Machine.vi"("State(s) in (\"\")"=w251) -> ("States Out"=w250:string)  [unwired: 14 in]
        n81 = case shown="\"Close\", \"Closed\"" w245 {
          tunnel: w249 -> [w257 w272 w283 w296 w309]
          tunnel: [w259 w273 w285 w298 w311] -> w248
          tunnel: w246 -> [w258 w270 w284 w297 w310]
          frame "Open", "Standard", Default {
            w252 = T5."Standard" ("State")
            n82 = property class="VI"(reference=w258, error in=w257) -> (reference out=w255:refnum<vi>, error out=w256:errorcluster, "FP.State"=w254:T5)
            n83 = Not Equal?(x=w254, y=w252) -> (x != y?=w253:bool)
            n84 = case shown="True" w253 {
              tunnel: [w263 w265] -> w259
              tunnel: w256 -> [w262 w265]
              tunnel: w255 -> [w261 _]
              tunnel: w252 -> [w260 _]
              frame True {
                n85 = invoke class="VI" method="FP.Open"(reference=w261, error in=w262, "Activate"=TRUE, "State"=w260) -> (error out=w263:errorcluster)  [unwired: 1 in, 4 out]
              }
              frame False {
              }
            }
          }
          frame "Close", "Closed" {
            n86 = property class="VI"(reference=w270, error in=w272) -> (reference out=w269:refnum<vi>, error out=w271:errorcluster, "FP.State"=w267:T5)
            n87 = Not Equal?(x=w267, y=T5."Closed" ("Front Panel Window:State")) -> (x != y?=w266:bool)
            n88 = case shown="False" w266 {
              tunnel: [w274 w277] -> w273
              tunnel: w271 -> [w274 w276]
              tunnel: w269 -> [_ w275]
              frame False {
              }
              frame True {
                n89 = invoke class="VI" method="FP.Close"(reference=w275, error in=w276) -> (error out=w277:errorcluster)  [unwired: 1 in, 2 out]
              }
            }
          }
          frame "Hidden", "Hide" {
            w278 = T5."Hidden" ("State")
            n90 = property class="VI"(reference=w284, error in=w283) -> (reference out=w281:refnum<vi>, error out=w282:errorcluster, "FP.State"=w280:T5)
            n91 = Not Equal?(x=w280, y=w278) -> (x != y?=w279:bool)
            n92 = case shown="True" w279 {
              tunnel: [w289 w290] -> w285
              tunnel: w282 -> [w288 w290]
              tunnel: w281 -> [w287 _]
              tunnel: w278 -> [w286 _]
              frame True {
                n93 = invoke class="VI" method="FP.Open"(reference=w287, error in=w288, "State"=w286) -> (error out=w289:errorcluster)  [unwired: 2 in, 4 out]
              }
              frame False {
              }
            }
          }
          frame "Minimize", "Minimized" {
            w291 = T5."Minimized" ("State")
            n94 = property class="VI"(reference=w297, error in=w296) -> (reference out=w294:refnum<vi>, error out=w295:errorcluster, "FP.State"=w293:T5)
            n95 = Not Equal?(x=w293, y=w291) -> (x != y?=w292:bool)
            n96 = case shown="True" w292 {
              tunnel: [w302 w303] -> w298
              tunnel: w295 -> [w301 w303]
              tunnel: w294 -> [w300 _]
              tunnel: w291 -> [w299 _]
              frame True {
                n97 = invoke class="VI" method="FP.Open"(reference=w300, error in=w301, "State"=w299) -> (error out=w302:errorcluster)  [unwired: 2 in, 4 out]
              }
              frame False {
              }
            }
          }
          frame "Maximize", "Maximized" {
            w304 = T5."Maximized" ("State")
            n98 = property class="VI"(reference=w310, error in=w309) -> (reference out=w307:refnum<vi>, error out=w308:errorcluster, "FP.State"=w306:T5)
            n99 = Not Equal?(x=w306, y=w304) -> (x != y?=w305:bool)
            n100 = case shown="True" w305 {
              tunnel: [w315 w316] -> w311
              tunnel: w308 -> [w314 w316]
              tunnel: w307 -> [w313 _]
              tunnel: w304 -> [w312 _]
              frame True {
                n101 = invoke class="VI" method="FP.Open"(reference=w313, error in=w314, "State"=w312) -> (error out=w315:errorcluster)  [unwired: 2 in, 4 out]
              }
              frame False {
              }
            }
          }
        }
      }
      frame "---------- Macro ----------" {
        # "#CSM \"Category Seperator\"\nDo not put any code in this frame."
        n102 = call <vilib>:"Add State(s) to Queue__JKI_lib_State_Machine.vi"("State(s) in (\"\")"=w321) -> ("States Out"=w320:string)  [unwired: 14 in]
      }
      frame "Macro: Initialize" {
        w323 = "Data: Initialize\nInitialize Core Data\nEvents: Register\nUI: Initialize\nUI: Front Panel State >> Open"  # Data: Initialize Initialize Core Data Events: Register UI: Initialize UI: Front Panel State >> Open
        # "#CSM \"Macro: Initialize\"\nInitialization Macro (This is called once, when the VI starts)"
        n103 = call <vilib>:"Add State(s) to Queue__JKI_lib_State_Machine.vi"("State(s) in Front (\"\")"=w323, "State(s) in (\"\")"=w327) -> ("States Out"=w326:string)  [unwired: 13 in]
      }
      frame "Macro: Exit" {
        # "#CSM \"Macro: Exit\"\nExit Macro (This is called once, when the VI exits)"
        n104 = Unbundle By Name(w336) -> ("Core.Close Panel on Exit?"=w335:bool)
        n105 = Select(t="UI: Front Panel State >> Close", s=w335, f="") -> (s? t:f=w332:string)
        n106 = call <vilib>:"Add State(s) to Queue__JKI_lib_State_Machine.vi"("State(s) in Front (\"\")"="//Exit Sub-Modules ", "State(s) in (\"\")"=w332, "State(s) at Back (\"\")"="Data: Cleanup\nEvents: Unregister\nExit") -> ("States Out"=w330:string)  [unwired: 12 in]
        n107 = call <vilib>:"Add State(s) to Queue__JKI_lib_State_Machine.vi"("State(s) in Front (\"\")"=w330, "State(s) in (\"\")"=w339) -> ("States Out"=w338:string)  [unwired: 13 in]
      }
      frame "---------- API ----------" {
        # "#CSM \"Category Seperator\"\nDo not put any code in this frame."
      }
      frame "API: Button Click" {
        # "#CSM-Example Step3"
        # "#CSM API Example\nCopy/Rename this case for your own API"
      }
    }
  }
